vi "Demo_Simple.vi"() -> ()   [LabVIEW 2018]
panel:
  out "error out":errorcluster
  in  "Reset at Init":bool=TRUE
  in  "Motor":bool
  in  "Input":dbl
  in  "Case":T1(ring)
  out "Output":dbl
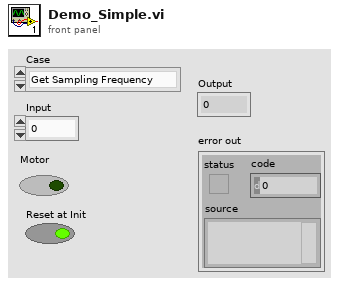
[diagram p1: front panel]
types:
  T1 = enum16{"Get Sampling Frequency", "Get Scan Frequency", "Get Scan Amplitude", "Set Sampling Frequency", "Set Scan Frequency", "Set Scan Amplitunde", "Motor ON/OFF"}
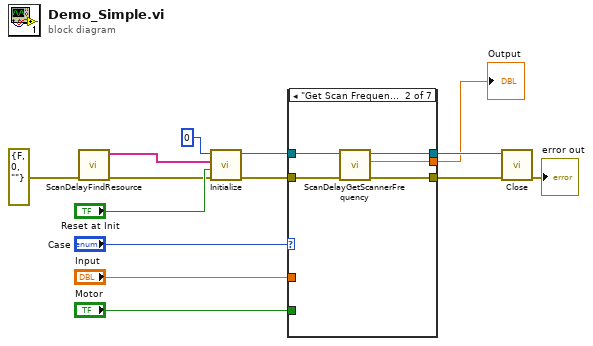
[diagram p0: block diagram]
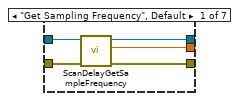
[diagram p2: hidden frame]
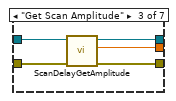
[diagram p3: hidden frame]
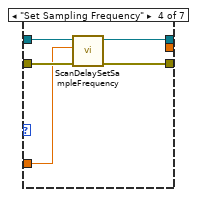
[diagram p4: hidden frame]
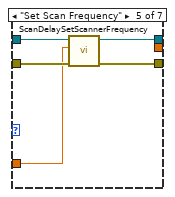
[diagram p5: hidden frame]
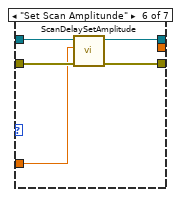
[diagram p6: hidden frame]
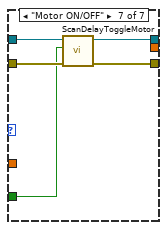
[diagram p7: hidden frame]
diagram:
  n1 = call "ScanDelayFindResource.vi"("error in (no error)"=errorcluster {"status"=FALSE, "code"=0, "source"=""}) -> ("error out"=w7:errorcluster, "resource array"=w6:string[])  [unwired: 8 in, 1 out]
  n2 = call "Initialize.vi"("error in (no error)"=w7, "Reset (True)"="Reset at Init", "resource array"=w6, "Resource"=0) -> ("VISA Error Out"=w14:errorcluster, "VISA  name out"=w11:refnum<visa-resource-name>)  [unwired: 5 in, 1 out]
  n3 = case shown="\"Get Scan Frequency\"" "Case" {
    tunnel: w14 -> [w19 w23 w29 w34 w39 w44 w49]
    tunnel: [w18 w22 w26 w32 w36 w41 w48] -> w13
    tunnel: [w17 w20 w27 w31 w37 w42 w47] -> w12
    tunnel: w11 -> [w16 w24 w28 w33 w38 w43 w46]
    tunnel: [w15 w21 w25 _ _ _ _] -> w9
    tunnel: "Input" -> [_ _ _ w30 w35 w40 _]
    tunnel: "Motor" -> [_ _ _ _ _ _ w45]
    frame "Get Sampling Frequency", Default {
      n4 = call "ScanDelayGetSampleFrequency.vi"("error in (no error)"=w19, "VISA resource name in"=w16) -> ("error out"=w18:errorcluster, "value"=w15:dbl, "VISA resource name out"=w17:refnum<visa-resource-name>)  [unwired: 7 in]
    }
    frame "Get Scan Frequency" {
      n5 = call "ScanDelayGetScannerFrequency.vi"("error in (no error)"=w23, "VISA resource name in"=w24) -> ("error out"=w22:errorcluster, "value"=w21:dbl, "VISA resource name out"=w20:refnum<visa-resource-name>)  [unwired: 7 in]
    }
    frame "Get Scan Amplitude" {
      n6 = call "ScanDelayGetAmplitude.vi"("error in (no error)"=w29, "VISA resource name in"=w28) -> ("error out"=w26:errorcluster, "value"=w25:dbl, "VISA resource name out"=w27:refnum<visa-resource-name>)  [unwired: 7 in]
    }
    frame "Set Sampling Frequency" {
      n7 = call "ScanDelaySetSampleFrequency.vi"("error in (no error)"=w34, "value"=w30, "VISA resource name in"=w33) -> ("error out"=w32:errorcluster, "VISA resource name out"=w31:refnum<visa-resource-name>)  [unwired: 7 in]
    }
    frame "Set Scan Frequency" {
      n8 = call "ScanDelaySetScannerFrequency.vi"("error in (no error)"=w39, "value"=w35, "VISA resource name in"=w38) -> ("error out"=w36:errorcluster, "VISA resource name out"=w37:refnum<visa-resource-name>)  [unwired: 7 in]
    }
    frame "Set Scan Amplitunde" {
      n9 = call "ScanDelaySetAmplitude.vi"("error in (no error)"=w44, "value"=w40, "VISA resource name in"=w43) -> ("error out"=w41:errorcluster, "VISA resource name out"=w42:refnum<visa-resource-name>)  [unwired: 7 in]
    }
    frame "Motor ON/OFF" {
      n10 = call "ScanDelayToggleMotor.vi"("error in (no error)"=w49, "value"=w45, "VISA resource name in"=w46) -> ("error out"=w48:errorcluster, "VISA resource name out"=w47:refnum<visa-resource-name>)  [unwired: 7 in]
    }
  }
  "Output" <- w9
  n11 = call "Close.vi"("error in (no error)"=w13, "VISA resource name"=w12) -> ("error out"=→"error out":errorcluster)  [unwired: 9 in]
